vi "_Check Voltages.vi"(6 "Unit":bool, 7 "SGInput":dbl[](array[numeric]), 8 "ADC Table":T3[](array[typedef]), 9 "ADC Values":i32[](array[numeric]), 10 "VoltageInput":dbl[](array[numeric]), 11 "Reference":T1) -> (0 "Source 2 Type:":T2 items=["None", "ESI", "APCI", "APPI", "MicroSpray"], 1 "Source 1 Type:":T2 items=["None", "ESI", "APCI", "APPI", "MicroSpray"], 2 "SVG OK":bool, 3 "Voltage OK":bool, 4 "Pressure":string[][](array[string]), 5 "DC OK":bool)   [LabVIEW 2018]
uses:
  Type/_RT Configuration 2.ctl
  Type/_Source Type.ctl
  Type/_Model Family.ctl
  <vilib>/Utility/miscctls.llb/LVRowAndColumnTypeDef.ctl
  Configuration/_Global Configuration.vi
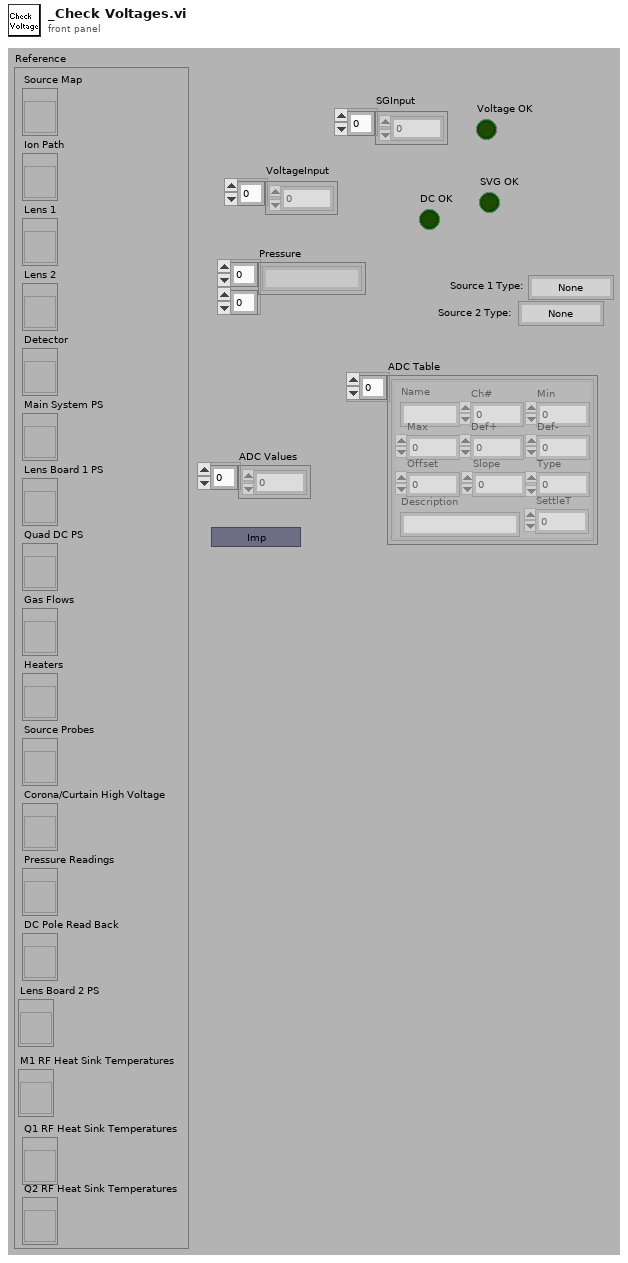
[diagram p1: front panel]
types:
  T1 = cluster{"Source Map":refnum<vi>, "Ion Path":refnum<vi>, "Lens 1":refnum<vi>, "Lens 2":refnum<vi>, "Detector":refnum<vi>, "Main System PS":refnum<vi>, "Lens Board 1 PS":refnum<vi>, "Quad DC PS":refnum<vi>, "Gas Flows":refnum<vi>, "Heaters":refnum<vi>, "Source Probes":refnum<vi>, "Corona/Curtain High Voltage":refnum<vi>, "Pressure Readings":refnum<vi>, "DC Pole Read Back":refnum<vi>, "Lens Board 2 PS":refnum<vi>, "M1 RF Heat Sink Temperatures":refnum<vi>, "Q1 RF Heat Sink Temperatures":refnum<vi>, "Q2 RF Heat Sink Temperatures":refnum<vi>}
  T2 = typedef "_Source Type.ctl" = i8
  T3 = typedef "_RT Configuration 2.ctl" = cluster{"Name":string, "Ch#":u8, "Min":dbl, "Max":dbl, "Def+":dbl, "Def-":dbl, "Offset":dbl, "Slope":dbl, "Type":u8, "Description":string, "SettleT":dbl}
  T4 = typedef "LVRowAndColumnTypeDef.ctl" = cluster{"Row":i32, "Column":i32}
  T5 = typedef "_Model Family.ctl" = u16
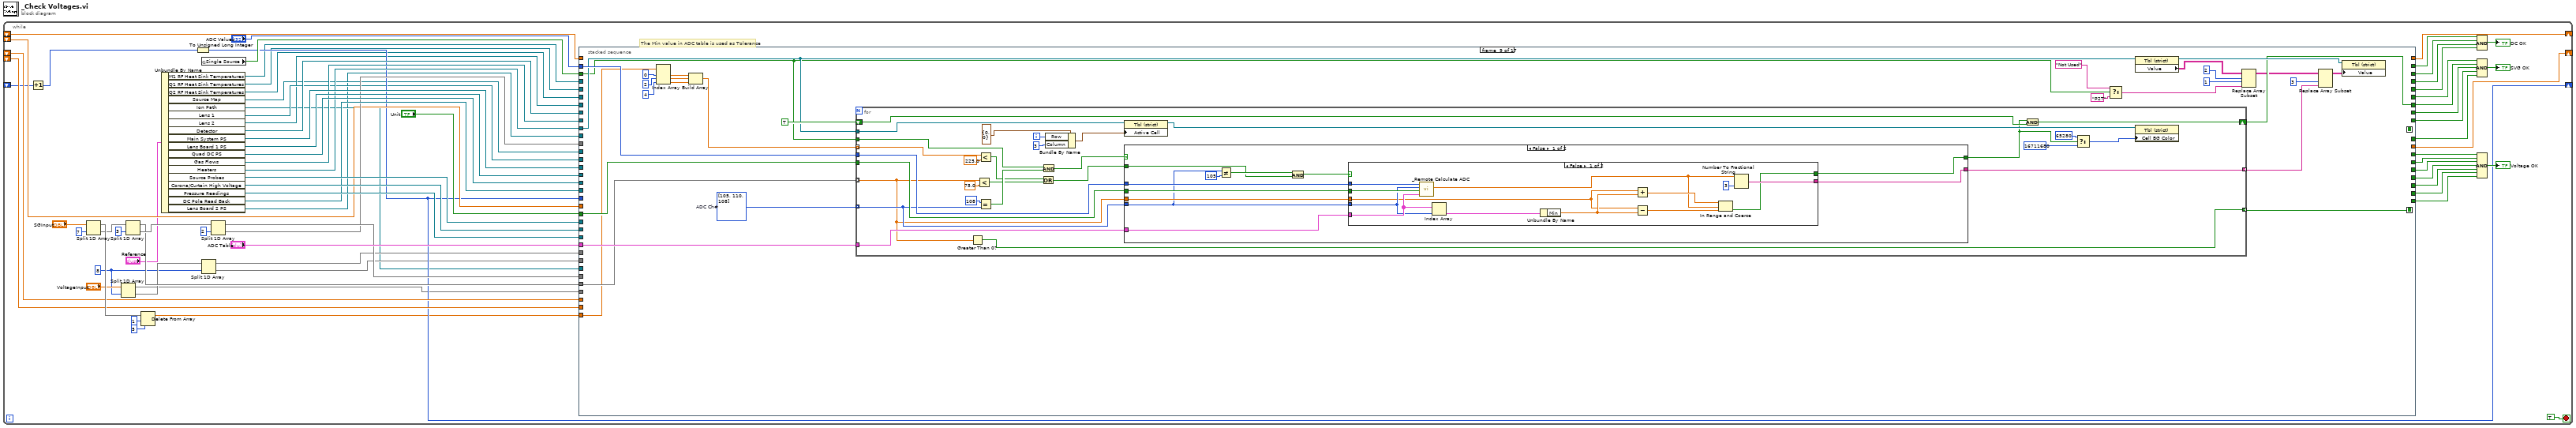
[diagram p0: block diagram]
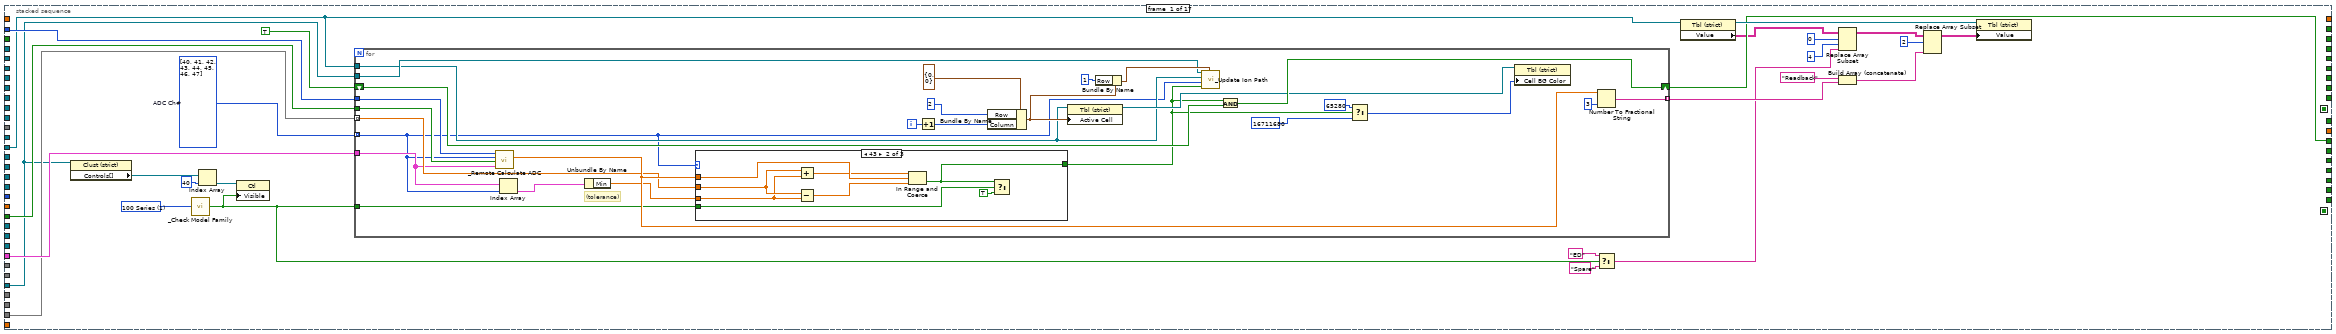
[diagram p2: hidden frame]
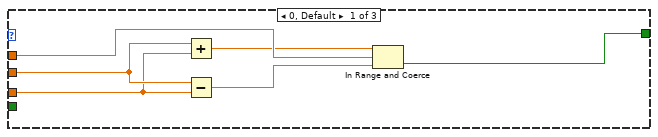
[diagram p3: hidden frame]
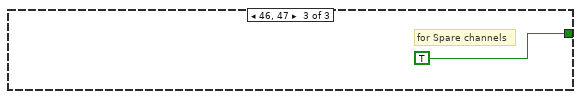
[diagram p4: hidden frame]
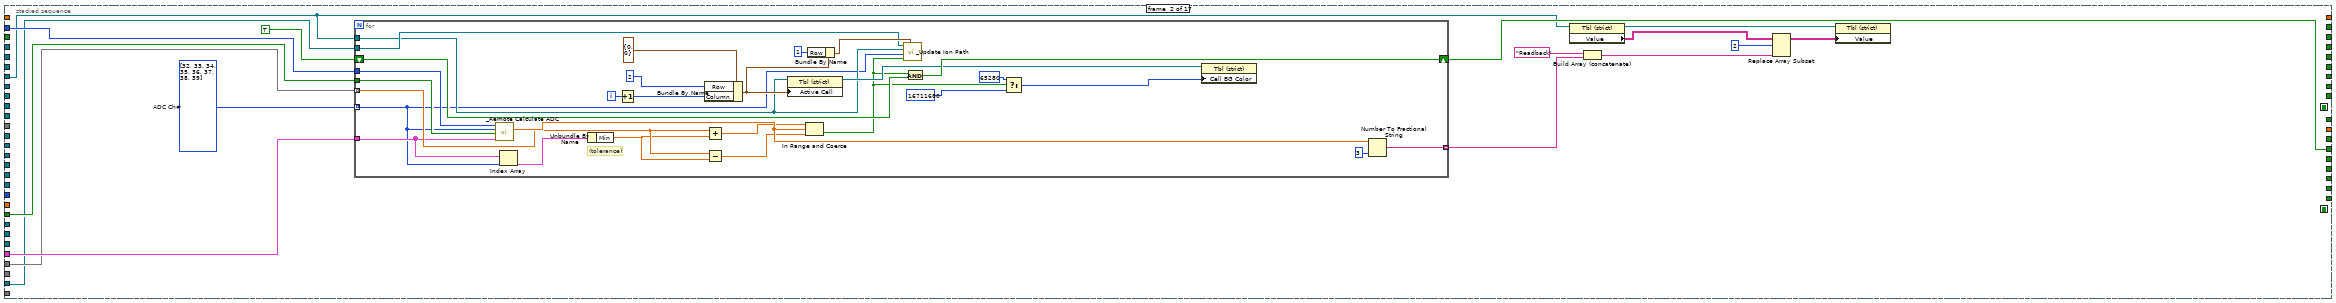
[diagram p5: hidden frame]
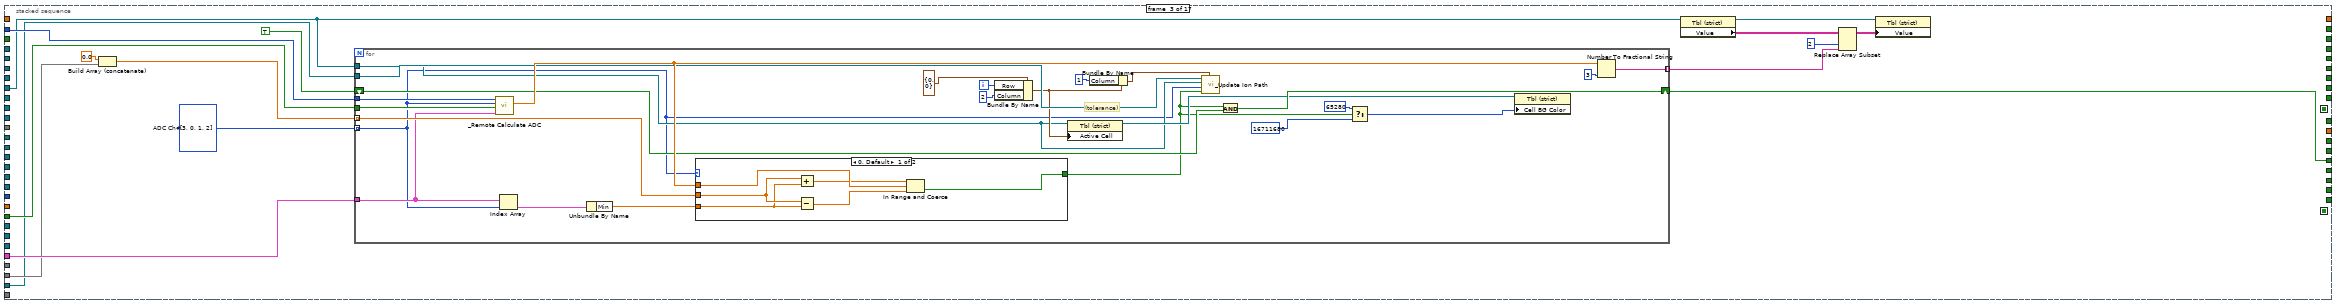
[diagram p6: hidden frame]
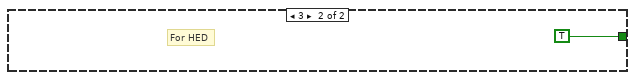
[diagram p7: hidden frame]
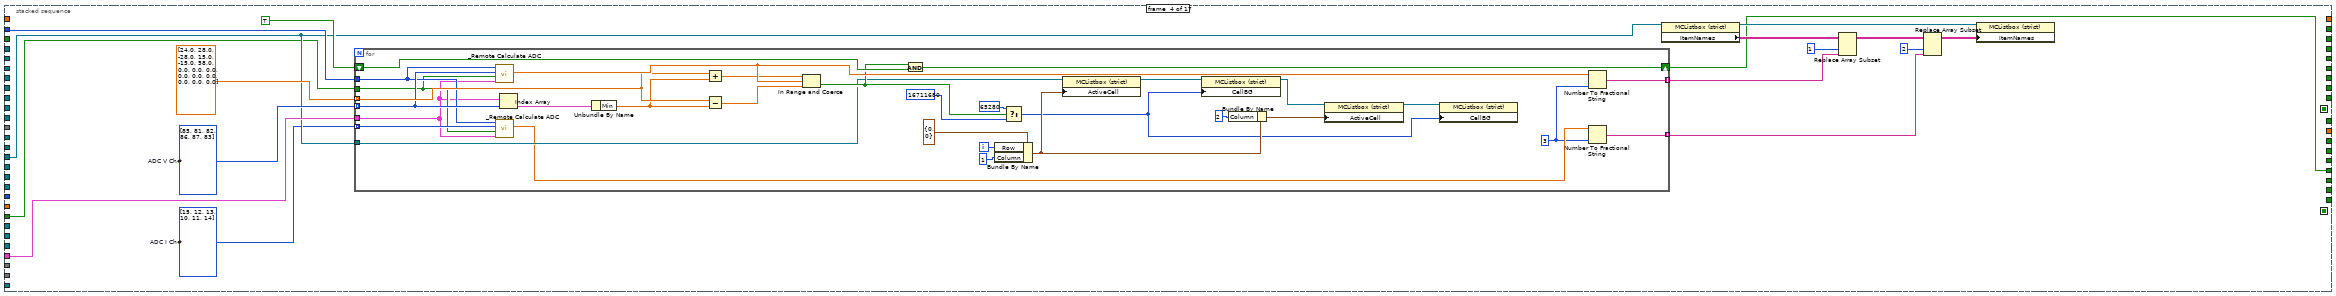
[diagram p8: hidden frame]
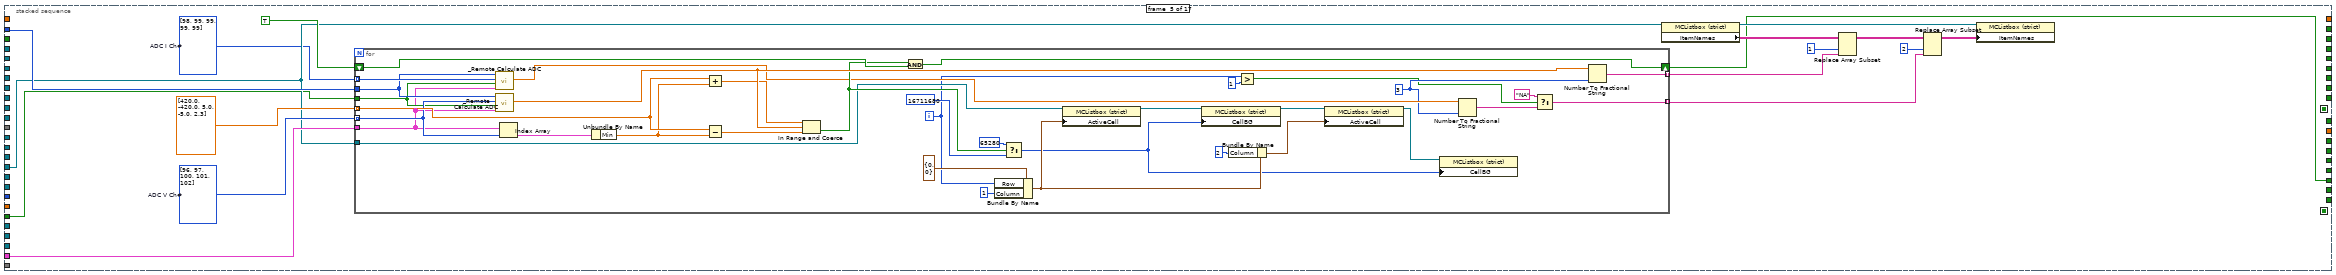
[diagram p9: hidden frame]
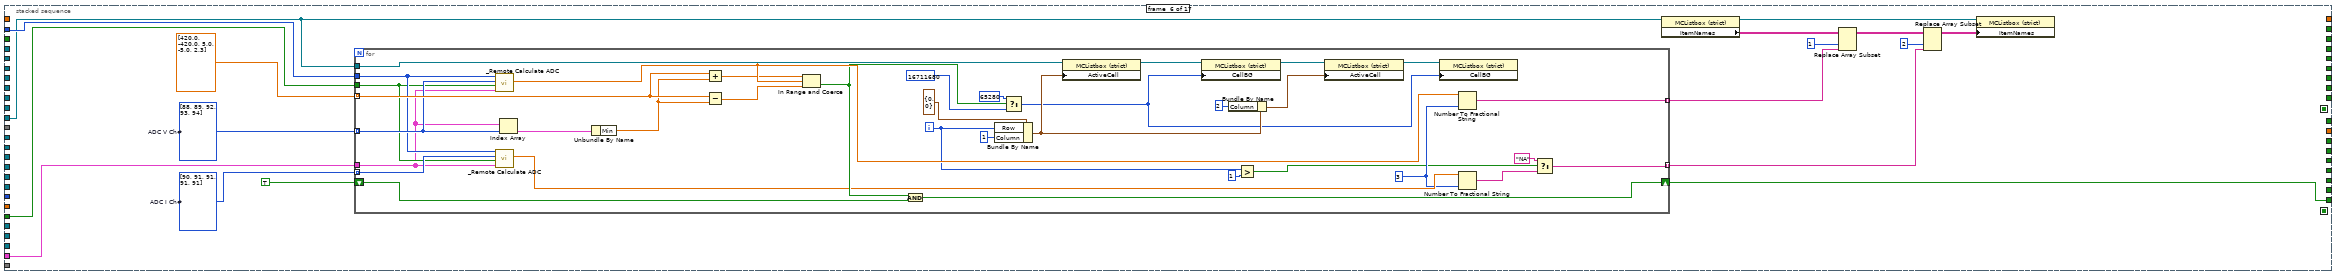
[diagram p10: hidden frame]
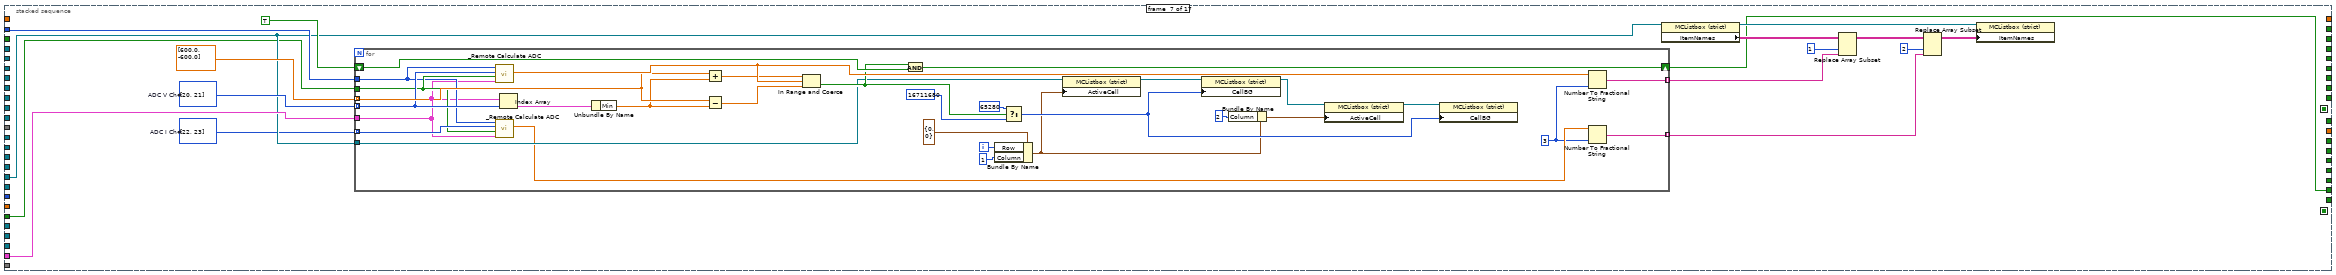
[diagram p11: hidden frame]
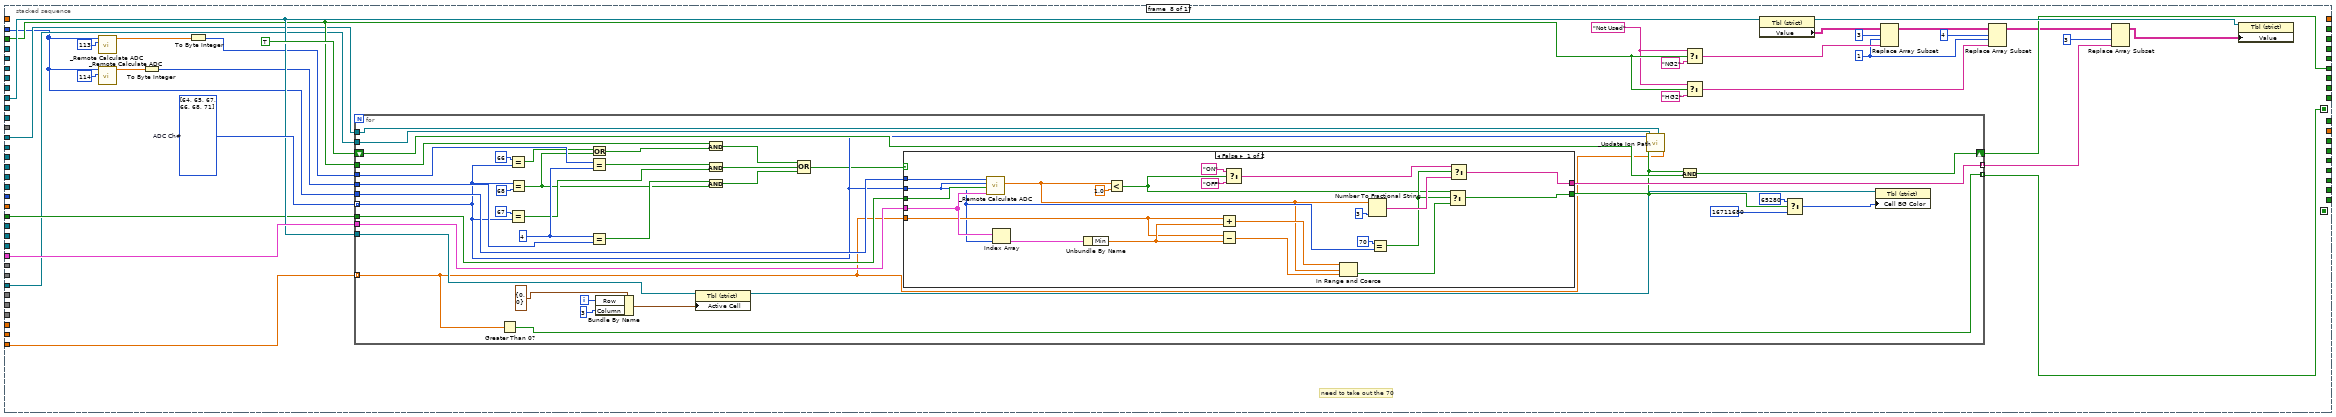
[diagram p12: hidden frame]
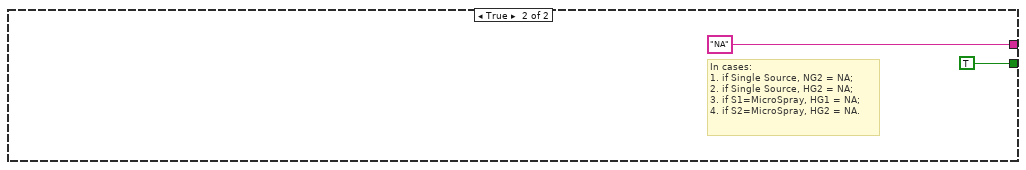
[diagram p13: hidden frame]
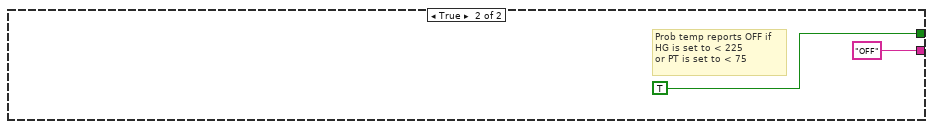
[diagram p14: hidden frame]
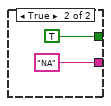
[diagram p15: hidden frame]
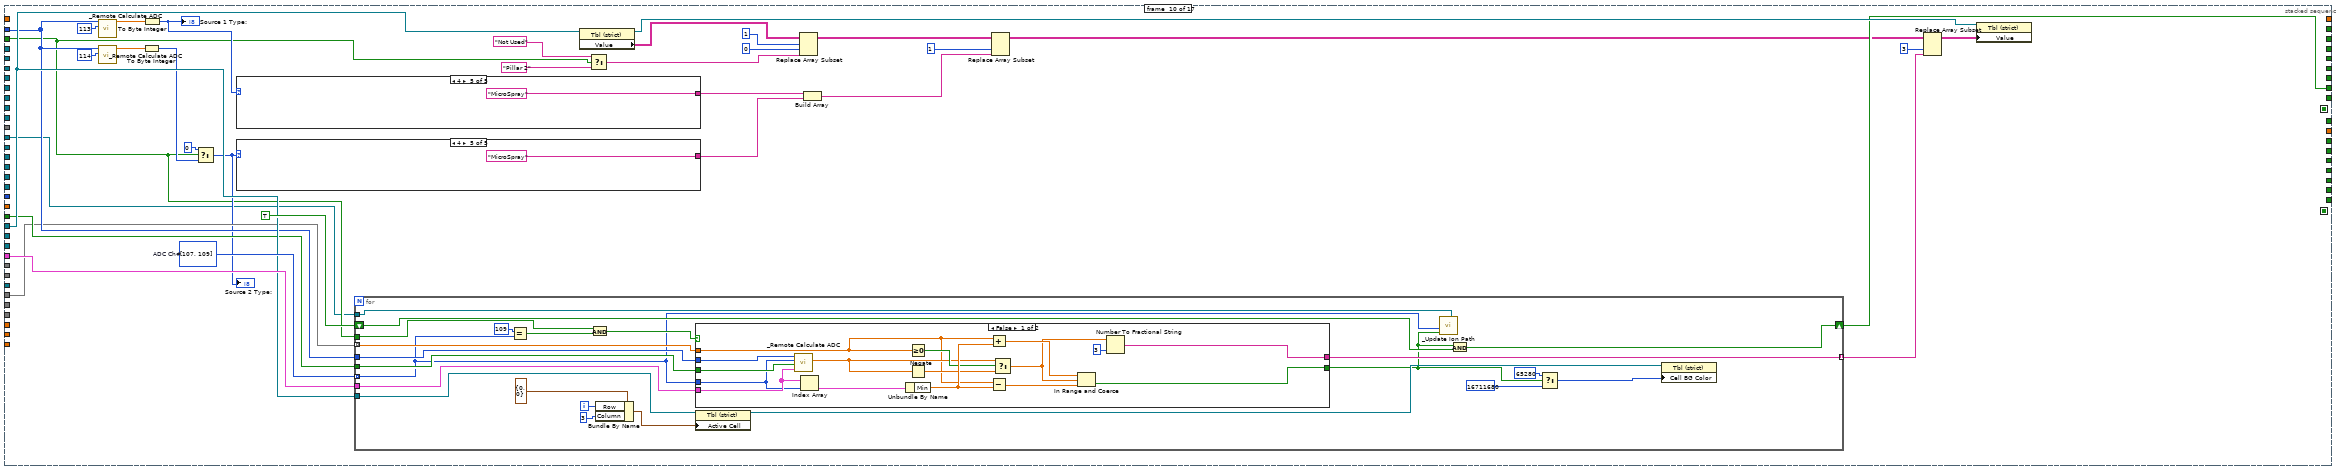
[diagram p16: hidden frame]
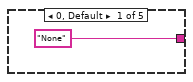
[diagram p17: hidden frame]
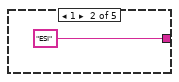
[diagram p18: hidden frame]
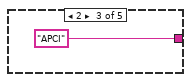
[diagram p19: hidden frame]
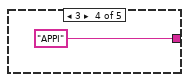
[diagram p20: hidden frame]
diagram:
  n1 = while {
    shift-right: [w35] -> _
    shift-left: _ -> [w34]
    shift-left: _ -> [w31]
    shift-right: [w33] -> _
    shift-left: _ -> [w32]
    shift-left: _ -> [w30]
    shift-right: [w27] -> _
    shift-left: _ -> [w29]
    stop <- TRUE stop-if-true
    w21 = 8 ("index")
    # "The Min value in ADC table is used as Tolerance"
    n2 = Increment(x=w29) -> (x+1=w28:u32)
    n3 = Split 1D Array(array="SGInput", index=7) -> (first subarray=w45:dbl[], second subarray=w43:dbl[])
    n4 = Split 1D Array(array="VoltageInput", index=w21) -> (first subarray=w20:dbl[], second subarray=w23:dbl[])
    n5 = Split 1D Array(array=w43, index=3) -> (first subarray=w40:dbl[], second subarray=w41:dbl[])
    n6 = Delete From Array(array=w45, length=1, index=5) -> (array with subset deleted=w3:dbl[])  [unwired: 1 out]
    n7 = Unbundle By Name("Reference") -> ("M1 RF Heat Sink Temperatures"=w11:refnum<vi>, "Q1 RF Heat Sink Temperatures"=w10:refnum<vi>, "Q2 RF Heat Sink Temperatures"=w9:refnum<vi>, "Source Map"=w15:refnum<vi>, "Ion Path"=w16:refnum<vi>, "Lens 1"=w26:refnum<vi>, "Lens 2"=w25:refnum<vi>, "Detector"=w71:refnum<vi>, "Main System PS"=w70:refnum<vi>, "Lens Board 1 PS"=w69:refnum<vi>, "Quad DC PS"=w68:refnum<vi>, "Gas Flows"=w60:refnum<vi>, "Heaters"=w59:refnum<vi>, "Source Probes"=w58:refnum<vi>, "Corona/Curtain High Voltage"=w57:refnum<vi>, "Pressure Readings"=w56:refnum<vi>, "DC Pole Read Back"=w49:refnum<vi>, "Lens Board 2 PS"=w13:refnum<vi>)
    n8 = To Unsigned Long Integer(number=w28) -> (unsigned 32bit integer=w27:u32)
    n9 = global read "_Global Configuration.vi" "Single Source"() -> (w37:bool)
    n10 = Split 1D Array(array=w23, index=w21) -> (first subarray=w19:dbl[], second subarray=w18:dbl[])
    n11 = Split 1D Array(array=w41, index=2) -> (first subarray=w39:dbl[], second subarray=w38:dbl[])
    n12 = stacked-sequence {
      seq-local: [_ _ _ _ _ _ _ _ w528 _ _ _ _ _ _ _ _] -> [_ _ _ _ _ _ _ _ _ _ _ _ _ _ _ _ w955]
      seq-local: [_ _ _ _ _ _ _ w443 _ _ _ _ _ _ _ _ _] -> [_ _ _ _ _ _ _ _ _ _ _ _ _ _ _ _ w952]
      tunnel: w71 -> [_ _ w196 _ _ _ _ _ _ _ _ _ _ _ _ _ _]
      tunnel: w70 -> [_ _ _ w240 _ _ _ _ _ _ _ _ _ _ _ _ _]
      tunnel: w69 -> [_ _ _ _ w288 _ _ _ _ _ _ _ _ _ _ _ _]
      tunnel: w68 -> [_ _ _ _ _ _ w392 _ _ _ _ _ _ _ _ _ _]
      tunnel: "ADC Values" -> [w97 w155 w199 w247 w295 w347 w399 w436 w555 w638 w713 w765 w830 w859 w890 w921 _]
      tunnel: "ADC Table" -> [w96 w154 w198 w246 w294 w346 w398 w464 w554 w646 w712 w764 w829 w858 w889 w920 _]
      tunnel: [_ _ w190 _ _ _ _ _ _ _ _ _ _ _ _ _ _] -> w65
      tunnel: [_ _ _ w239 _ _ _ _ _ _ _ _ _ _ _ _ _] -> w64
      tunnel: [_ _ _ _ w287 _ _ _ _ _ _ _ _ _ _ _ _] -> w63
      tunnel: [_ _ _ _ _ _ w391 _ _ _ _ _ _ _ _ _ _] -> w62
      tunnel: w60 -> [_ _ _ _ _ _ _ w459 _ _ _ _ _ _ _ _ _]
      tunnel: [_ _ _ _ _ _ _ w458 _ _ _ _ _ _ _ _ _] -> w55
      tunnel: w59 -> [_ _ _ _ _ _ _ _ w548 _ _ _ _ _ _ _ _]
      tunnel: [_ _ _ _ _ _ _ _ w547 _ _ _ _ _ _ _ _] -> w54
      tunnel: w58 -> [_ _ _ _ _ _ _ _ _ w642 _ _ _ _ _ _ _]
      tunnel: [_ _ _ _ _ _ _ _ _ w641 _ _ _ _ _ _ _] -> w53
      tunnel: w57 -> [_ _ _ _ _ _ _ _ _ _ w707 _ _ _ _ _ _]
      tunnel: [_ _ _ _ _ _ _ _ _ _ w706 _ _ _ _ _ _] -> w52
      tunnel: w56 -> [_ _ _ _ _ _ _ _ _ _ _ w760 _ _ _ _ _]
      tunnel: [_ _ _ _ _ _ _ _ _ _ _ w761 _ _ _ _ _] -> w51
      tunnel: [_ _ _ _ _ _ _ _ _ _ _ _ w824 _ _ _ _] -> w8
      tunnel: w49 -> [_ _ _ _ _ _ _ _ _ _ _ _ w821 _ _ _ _]
      tunnel: "Unit" -> [w92 w149 w189 w238 w286 w340 w390 w457 w546 w631 w705 w757 w823 w853 w884 w916 _]
      tunnel: w3 -> [_ _ _ _ _ _ _ w456 w536 _ _ _ _ _ _ _ _]
      tunnel: w40 -> [_ _ _ _ _ _ _ _ w545 _ _ _ _ _ _ _ _]
      tunnel: w39 -> [_ _ _ _ _ _ _ _ _ w626 _ _ _ _ _ _ _]
      tunnel: w38 -> [_ _ _ _ _ _ _ _ _ _ w702 _ _ _ _ _ _]
      tunnel: w37 -> [_ _ _ _ _ _ _ w455 w538 w615 _ _ _ _ _ _ _]
      tunnel: [_ _ _ _ _ _ _ _ _ _ _ w755 _ _ _ _ _] -> w35
      tunnel: w34 -> [_ _ _ _ _ _ _ _ _ _ _ w754 _ _ _ _ _]
      tunnel: [_ _ _ _ _ _ _ _ _ _ _ w753 _ _ _ _ _] -> w33
      tunnel: w32 -> [_ _ _ _ _ _ _ _ _ _ _ w752 _ _ _ _ _]
      tunnel: w31 -> [_ _ _ _ _ _ _ _ _ _ _ w751 _ _ _ _ _]
      tunnel: w30 -> [_ _ _ _ _ _ _ _ _ _ _ w750 _ _ _ _ _]
      tunnel: w27 -> [_ _ _ _ _ _ _ _ _ _ _ w747 _ _ _ _ _]
      tunnel: w26 -> [w91 _ _ _ _ _ _ _ _ _ _ _ _ _ _ _ _]
      tunnel: w25 -> [_ w142 _ _ _ _ _ _ _ _ _ _ _ _ _ _ _]
      tunnel: [w86 _ _ _ _ _ _ _ _ _ _ _ _ _ _ _ _] -> w24
      tunnel: w20 -> [w85 _ _ _ _ _ _ _ _ _ _ _ _ _ _ _ _]
      tunnel: w19 -> [_ w143 _ _ _ _ _ _ _ _ _ _ _ _ _ _ _]
      tunnel: w18 -> [_ _ w187 _ _ _ _ _ _ _ _ _ _ _ _ _ _]
      tunnel: [_ w144 _ _ _ _ _ _ _ _ _ _ _ _ _ _ _] -> w17
      tunnel: w16 -> [w75 w141 w185 _ _ _ _ w441 _ _ w700 _ _ _ _ _ _]
      tunnel: w15 -> [_ _ _ _ _ _ _ w442 _ w614 w699 _ _ _ _ _ w958]
      tunnel: w13 -> [_ _ _ _ _ w334 _ _ _ _ _ _ _ _ _ _ _]
      tunnel: [_ _ _ _ _ w333 _ _ _ _ _ _ _ _ _ _ _] -> w12
      tunnel: w11 -> [_ _ _ _ _ _ _ _ _ _ _ _ _ w850 _ _ _]
      tunnel: w10 -> [_ _ _ _ _ _ _ _ _ _ _ _ _ _ w881 _ _]
      tunnel: w9 -> [_ _ _ _ _ _ _ _ _ _ _ _ _ _ _ w913 _]
      tunnel: [_ _ _ _ _ _ _ _ _ _ _ _ _ w849 _ _ _] -> w6
      tunnel: [_ _ _ _ _ _ _ _ _ _ _ _ _ _ w880 _ _] -> w5
      tunnel: [_ _ _ _ _ _ _ _ _ _ _ _ _ _ _ w911 _] -> w4
      frame #0 {
        w77 = T5 1 items=["8080 Series", "100 Series", "200 Series", "300 Series", "Other Series"] ("Model Family (100)")
        w98 = u8[] [40, 41, 42, 43, 44, 45, 46, 47]  # ADC Ch#
        n13 = property class="Clust (strict)"(reference=w75) -> ("Controls[]"=w76:refnum<vi>[])  [unwired: 1 in, 2 out]
        n14 = call "_Check Model Family.vi"("Model Family (100)"=w77) -> ("Yes"=w72:bool)
        n15 = Index Array(array=w76, index=40) -> (element=w73:refnum<vi>)
        n16 = property class="Ctl"(reference=w73, "Visible"=w72) -> ()  [unwired: 1 in, 2 out]
        n17 = for {
          tunnel: w98 -> [w100] mode=indexing
          tunnel: w85 -> [w122] mode=indexing
          tunnel: w97 -> [w125]
          tunnel: w96 -> [w112]
          shift-right: [w120] -> w86
          shift-left: TRUE -> [w121]
          tunnel: w91 -> [w101]
          tunnel: [w114] -> w88 mode=indexing
          tunnel: w92 -> [w113]
          tunnel: w75 -> [w102]
          tunnel: w72 -> [w99]
          i -> [w108]
          # "(tolerance)"
          n18 = call "_Remote Calculate ADC.vi"("ADC Table"=w112, "Unit"=w113, "ADC Channel (64)"=w100, "ADC Values"=w125) -> ("User Value"=w123:dbl)  [unwired: 3 out]
          n19 = Index Array(array=w112, index=w100) -> (element=w111:T3)
          n20 = Unbundle By Name(w111) -> ("Min"=w110:dbl)
          n21 = case shown="43" w100 {
            tunnel: w123 -> [w131 w139 _]
            tunnel: w122 -> [w130 w138 _]
            tunnel: [w129 w133 TRUE] -> w106
            tunnel: w110 -> [w126 w135 _]
            tunnel: w99 -> [_ w134 _]
            frame 0, Default {
              n22 = Add(x=w130, y=w126) -> (x+y=w128:dbl)
              n23 = Subtract(x=w130, y=w126) -> (x-y=w127:dbl)
              n24 = In Range and Coerce(upper limit=w128, x=w131, lower limit=w127) -> (In Range?=w129:bool)  [unwired: 1 out]
            }
            frame 43 {
              n25 = Add(x=w138, y=w135) -> (x+y=w137:dbl)
              n26 = Subtract(x=w138, y=w135) -> (x-y=w136:dbl)
              n27 = In Range and Coerce(upper limit=w137, x=w139, lower limit=w136) -> (In Range?=w133:bool)  [unwired: 1 out]
              n28 = Select(t=w133, s=w134, f=TRUE) -> ()  [unwired: 1 out]
            }
            frame 46, 47 {
              # "for Spare channels"
            }
          }
          n29 = Increment(x=w108) -> (x+1=w107:i32)
          n30 = Bundle By Name(cluster=T4 {"Row"=0, "Column"=0} ("Active Cell:Active Cell"), "Row"=2 ("Column"), "Column"=w107) -> (w105:T4)
          n31 = property class="Tbl (strict)"(reference=w101, "Active Cell"=w105) -> (reference out=w116:refnum<vi>)  [unwired: 1 in, 1 out]
          n32 = Bundle By Name(cluster=w105, "Row"=1) -> (w104:T4)
          n33 = call "_Update Ion Path.vi"("Current Cell"=w104, "Voltage OK"=w106, "ADC Ch#"=w100, "Lens Table"=w101, "Ion Path"=w102) -> ()  [unwired: 2 in, 3 out]
          n34 = And(x=w106, y=w121) -> (x .and. y?=w120:bool)
          n35 = Select(t=u32 65280 ("Active Cell:Cell Background Color"), s=w106, f=u32 16711680 ("Active Cell:Cell Background Color")) -> (s? t:f=w115:u32)
          n36 = property class="Tbl (strict)"(reference=w116, "Cell BG Color"=w115) -> ()  [unwired: 1 in, 2 out]
          n37 = Number To Fractional String(number=w123, precision (6)=i16 3) -> (F-format string=w114:string)  [unwired: 2 out]
        }
        n38 = Select(t="ED", s=w72, f="Spare") -> (s? t:f=w78:string)
        n39 = property class="Tbl (strict)"(reference=w91) -> (reference out=w94:refnum<vi>, "Value"=w82:string[][])  [unwired: 1 in, 1 out]
        n40 = Replace Array Subset(array=w82, new element=w78, index (row)=0, index (col)=4 ("disabled index (col)")) -> (w81:string[][])
        n41 = Build Array (concatenate)("Readback", w88) -> (w87:string[])
        n42 = Replace Array Subset(array=w81, new element=w87, index (row)=2 ("disabled index (col)")) -> (w93:string[][])  [unwired: 1 in]
        n43 = property class="Tbl (strict)"(reference=w94, "Value"=w93) -> ()  [unwired: 1 in, 2 out]
      }
      frame #1 {
        w156 = u8[] [32, 33, 34, 35, 36, 37, 38, 39]  # ADC Ch#
        n44 = for {
          tunnel: w156 -> [w157] mode=indexing
          tunnel: w143 -> [w181] mode=indexing
          tunnel: w155 -> [w184]
          tunnel: w154 -> [w171]
          shift-right: [w179] -> w144
          shift-left: TRUE -> [w180]
          tunnel: w142 -> [w158]
          tunnel: [w173] -> w146 mode=indexing
          tunnel: w149 -> [w172]
          tunnel: w141 -> [w159]
          i -> [w167]
          # "(tolerance)"
          n45 = call "_Remote Calculate ADC.vi"("ADC Table"=w171, "Unit"=w172, "ADC Channel (64)"=w157, "ADC Values"=w184) -> ("User Value"=w182:dbl)  [unwired: 3 out]
          n46 = Index Array(array=w171, index=w157) -> (element=w170:T3)
          n47 = Unbundle By Name(w170) -> ("Min"=w169:dbl)
          n48 = Increment(x=w167) -> (x+1=w166:i32)
          n49 = Bundle By Name(cluster=T4 {"Row"=0, "Column"=0} ("Active Cell:Active Cell"), "Row"=2 ("Column"), "Column"=w166) -> (w161:T4)
          n50 = Add(x=w181, y=w169) -> (x+y=w165:dbl)
          n51 = Subtract(x=w181, y=w169) -> (x-y=w164:dbl)
          n52 = property class="Tbl (strict)"(reference=w158, "Active Cell"=w161) -> (reference out=w175:refnum<vi>)  [unwired: 1 in, 1 out]
          n53 = In Range and Coerce(upper limit=w165, x=w182, lower limit=w164) -> (In Range?=w163:bool)  [unwired: 1 out]
          n54 = Bundle By Name(cluster=w161, "Row"=1) -> (w160:T4)
          n55 = call "_Update Ion Path.vi"("Current Cell"=w160, "Voltage OK"=w163, "ADC Ch#"=w157, "Lens Table"=w158, "Ion Path"=w159) -> ()  [unwired: 2 in, 3 out]
          n56 = And(x=w163, y=w180) -> (x .and. y?=w179:bool)
          n57 = Select(t=u32 65280 ("Active Cell:Cell Background Color"), s=w163, f=u32 16711680 ("Active Cell:Cell Background Color")) -> (s? t:f=w174:u32)
          n58 = property class="Tbl (strict)"(reference=w175, "Cell BG Color"=w174) -> ()  [unwired: 1 in, 2 out]
          n59 = Number To Fractional String(number=w182, precision (6)=i16 3) -> (F-format string=w173:string)  [unwired: 2 out]
        }
        n60 = property class="Tbl (strict)"(reference=w142) -> (reference out=w152:refnum<vi>, "Value"=w151:string[][])  [unwired: 1 in, 1 out]
        n61 = Build Array (concatenate)("Readback", w146) -> (w145:string[])
        n62 = Replace Array Subset(array=w151, new element=w145, index (row)=2 ("disabled index (col)")) -> (w150:string[][])  [unwired: 1 in]
        n63 = property class="Tbl (strict)"(reference=w152, "Value"=w150) -> ()  [unwired: 1 in, 2 out]
      }
      frame #2 {
        w200 = u8[] [3, 0, 1, 2]  # ADC Ch#
        n64 = Build Array (concatenate)(0.0 ("element"), w187) -> (w186:dbl[])
        n65 = for {
          tunnel: w200 -> [w201] mode=indexing
          tunnel: w186 -> [w222] mode=indexing
          tunnel: w199 -> [w225]
          tunnel: w198 -> [w211]
          shift-right: [w220] -> w190
          shift-left: TRUE -> [w221]
          tunnel: w196 -> [w202]
          tunnel: [w213] -> w192 mode=indexing
          tunnel: w189 -> [w212]
          tunnel: w185 -> [w206]
          i -> [w210]
          # "(tolerance)"
          n66 = call "_Remote Calculate ADC.vi"("ADC Table"=w211, "Unit"=w212, "ADC Channel (64)"=w201, "ADC Values"=w225) -> ("User Value"=w223:dbl)  [unwired: 3 out]
          n67 = Index Array(array=w211, index=w201) -> (element=w209:T3)
          n68 = Unbundle By Name(w209) -> ("Min"=w208:dbl)
          n69 = case shown="0, Default" w201 {
            tunnel: w223 -> [w231 _]
            tunnel: w222 -> [w230 _]
            tunnel: [w229 TRUE] -> w207
            tunnel: w208 -> [w226 _]
            frame 0, Default {
              n70 = Add(x=w230, y=w226) -> (x+y=w228:dbl)
              n71 = Subtract(x=w230, y=w226) -> (x-y=w227:dbl)
              n72 = In Range and Coerce(upper limit=w228, x=w231, lower limit=w227) -> (In Range?=w229:bool)  [unwired: 1 out]
            }
            frame 3 {
              # "For HED"
            }
          }
          n73 = Bundle By Name(cluster=T4 {"Row"=0, "Column"=0} ("Active Cell:Active Cell"), "Row"=w210, "Column"=2) -> (w204:T4)
          n74 = property class="Tbl (strict)"(reference=w202, "Active Cell"=w204) -> (reference out=w215:refnum<vi>)  [unwired: 1 in, 1 out]
          n75 = Bundle By Name(cluster=w204, "Column"=1 ("Row")) -> (w203:T4)
          n76 = call "_Update Ion Path.vi"("Current Cell"=w203, "Voltage OK"=w207, "ADC Ch#"=w201, "Lens Table"=w202, "Ion Path"=w206) -> ()  [unwired: 2 in, 3 out]
          n77 = And(x=w207, y=w221) -> (x .and. y?=w220:bool)
          n78 = Select(t=u32 65280 ("Active Cell:Cell Background Color"), s=w207, f=u32 16711680 ("Active Cell:Cell Background Color")) -> (s? t:f=w214:u32)
          n79 = property class="Tbl (strict)"(reference=w215, "Cell BG Color"=w214) -> ()  [unwired: 1 in, 2 out]
          n80 = Number To Fractional String(number=w223, precision (6)=i16 3) -> (F-format string=w213:string)  [unwired: 2 out]
        }
        n81 = property class="Tbl (strict)"(reference=w196) -> (reference out=w195:refnum<vi>, "Value"=w194:string[][])  [unwired: 1 in, 1 out]
        n82 = Replace Array Subset(array=w194, new element=w192, index (col)=2 ("disabled index (col)")) -> (w191:string[][])  [unwired: 1 in]
        n83 = property class="Tbl (strict)"(reference=w195, "Value"=w191) -> ()  [unwired: 1 in, 2 out]
      }
      frame #3 {
        w237 = u8[] [15, 12, 13, 10, 11, 14]  # ADC I Ch#
        w249 = u8[] [85, 81, 82, 86, 87, 83]  # ADC V Ch#
        n84 = for {
          tunnel: w249 -> [w264] mode=indexing
          tunnel: dbl[] [24.0, 28.0, -28.0, 15.0, -15.0, 58.0, 0.0, 0.0, 0.0, 0.0, 0.0, 0.0, 0.0, 0.0, 0.0] ("VoltageInput 2") -> [w279] mode=indexing
          tunnel: w247 -> [w261]
          tunnel: w246 -> [w259]
          shift-right: [w277] -> w239
          shift-left: TRUE -> [w278]
          tunnel: w240 -> [w270]
          tunnel: [w268] -> w241 mode=indexing
          tunnel: w238 -> [w260]
          tunnel: w237 -> [w262] mode=indexing
          tunnel: [w256] -> w233 mode=indexing
          i -> [w271]
          w257 = i16 3 ("precision (6)")
          n85 = call "_Remote Calculate ADC.vi"("ADC Table"=w259, "Unit"=w260, "ADC Channel (64)"=w264, "ADC Values"=w261) -> ("User Value"=w280:dbl)  [unwired: 3 out]
          n86 = call "_Remote Calculate ADC.vi"("ADC Table"=w259, "Unit"=w260, "ADC Channel (64)"=w262, "ADC Values"=w261) -> ("User Value"=w258:dbl)  [unwired: 3 out]
          n87 = Index Array(array=w259, index=w264) -> (element=w265:T3)
          n88 = Unbundle By Name(w265) -> ("Min"=w263:dbl)
          n89 = Add(x=w279, y=w263) -> (x+y=w267:dbl)
          n90 = Subtract(x=w279, y=w263) -> (x-y=w266:dbl)
          n91 = In Range and Coerce(upper limit=w267, x=w280, lower limit=w266) -> (In Range?=w275:bool)  [unwired: 1 out]
          n92 = And(x=w275, y=w278) -> (x .and. y?=w277:bool)
          n93 = Bundle By Name(cluster=T4 {"Row"=0, "Column"=0} ("Active Cell:Active Cell"), "Row"=w271, "Column"=1) -> (w253:T4)
          n94 = Select(t=u32 65280 ("Active Cell:Cell Background Color"), s=w275, f=u32 16711680 ("Active Cell:Cell Background Color")) -> (s? t:f=w250:u32)
          n95 = property class="MCListbox (strict)"(reference=w270, "ActiveCell"=w253) -> (reference out=w269:refnum<vi>)  [unwired: 1 in, 1 out]
          n96 = property class="MCListbox (strict)"(reference=w269, "CellBG"=w250) -> (reference out=w254:refnum<vi>)  [unwired: 1 in, 1 out]
          n97 = Bundle By Name(cluster=w253, "Column"=2) -> (w251:T4)
          n98 = property class="MCListbox (strict)"(reference=w254, "ActiveCell"=w251) -> (reference out=w255:refnum<vi>)  [unwired: 1 in, 1 out]
          n99 = property class="MCListbox (strict)"(reference=w255, "CellBG"=w250) -> ()  [unwired: 1 in, 2 out]
          n100 = Number To Fractional String(number=w280, precision (6)=w257) -> (F-format string=w268:string)  [unwired: 2 out]
          n101 = Number To Fractional String(number=w258, precision (6)=w257) -> (F-format string=w256:string)  [unwired: 2 out]
        }
        n102 = property class="MCListbox (strict)"(reference=w240) -> (reference out=w244:refnum<vi>, "ItemNames"=w243:string[][])  [unwired: 1 in, 1 out]
        n103 = Replace Array Subset(array=w243, new element=w241, index (col)=1 ("disabled index (col)")) -> (w236:string[][])  [unwired: 1 in]
        n104 = Replace Array Subset(array=w236, new element=w233, index (col)=2 ("disabled index (col)")) -> (w235:string[][])  [unwired: 1 in]
        n105 = property class="MCListbox (strict)"(reference=w244, "ItemNames"=w235) -> ()  [unwired: 1 in, 2 out]
      }
      frame #4 {
        w282 = u8[] [98, 99, 99, 99, 99]  # ADC I Ch#
        w297 = u8[] [96, 97, 100, 101, 102]  # ADC V Ch#
        n106 = for {
          tunnel: w297 -> [w316] mode=indexing
          tunnel: dbl[] [420.0, -420.0, 5.0, -5.0, 2.3] ("VoltageInput 2") -> [w331] mode=indexing
          tunnel: w295 -> [w314]
          tunnel: w294 -> [w312]
          shift-right: [w329] -> w287
          shift-left: TRUE -> [w330]
          tunnel: w288 -> [w323]
          tunnel: [w321] -> w289 mode=indexing
          tunnel: w286 -> [w313]
          tunnel: w282 -> [w315] mode=indexing
          tunnel: [w304] -> w281 mode=indexing
          i -> [w309]
          w310 = i16 3 ("precision (6)")
          n107 = call "_Remote Calculate ADC.vi"("ADC Table"=w312, "Unit"=w313, "ADC Channel (64)"=w315, "ADC Values"=w314) -> ("User Value"=w311:dbl)  [unwired: 3 out]
          n108 = call "_Remote Calculate ADC.vi"("ADC Table"=w312, "Unit"=w313, "ADC Channel (64)"=w316, "ADC Values"=w314) -> ("User Value"=w332:dbl)  [unwired: 3 out]
          n109 = Index Array(array=w312, index=w316) -> (element=w318:T3)
          n110 = Unbundle By Name(w318) -> ("Min"=w317:dbl)
          n111 = Add(x=w331, y=w317) -> (x+y=w320:dbl)
          n112 = Subtract(x=w331, y=w317) -> (x-y=w319:dbl)
          n113 = In Range and Coerce(upper limit=w320, x=w332, lower limit=w319) -> (In Range?=w327:bool)  [unwired: 1 out]
          n114 = And(x=w327, y=w330) -> (x .and. y?=w329:bool)
          n115 = Bundle By Name(cluster=T4 {"Row"=0, "Column"=0} ("Active Cell:Active Cell"), "Row"=w309, "Column"=1) -> (w301:T4)
          n116 = Select(t=u32 65280 ("Active Cell:Cell Background Color"), s=w327, f=u32 16711680 ("Active Cell:Cell Background Color")) -> (s? t:f=w298:u32)
          n117 = property class="MCListbox (strict)"(reference=w323, "ActiveCell"=w301) -> (reference out=w322:refnum<vi>)  [unwired: 1 in, 1 out]
          n118 = property class="MCListbox (strict)"(reference=w322, "CellBG"=w298) -> (reference out=w302:refnum<vi>)  [unwired: 1 in, 1 out]
          n119 = Bundle By Name(cluster=w301, "Column"=2) -> (w299:T4)
          n120 = Greater?(x=w309, y=1) -> (0:w307:bool)
          n121 = property class="MCListbox (strict)"(reference=w302, "ActiveCell"=w299) -> (reference out=w303:refnum<vi>)  [unwired: 1 in, 1 out]
          n122 = property class="MCListbox (strict)"(reference=w303, "CellBG"=w298) -> ()  [unwired: 1 in, 2 out]
          n123 = Number To Fractional String(number=w311, precision (6)=w310) -> (F-format string=w306:string)  [unwired: 2 out]
          n124 = Select(t="NA", s=w307, f=w306) -> (s? t:f=w304:string)
          n125 = Number To Fractional String(number=w332, precision (6)=w310) -> (F-format string=w321:string)  [unwired: 2 out]
        }
        n126 = property class="MCListbox (strict)"(reference=w288) -> (reference out=w292:refnum<vi>, "ItemNames"=w291:string[][])  [unwired: 1 in, 1 out]
        n127 = Replace Array Subset(array=w291, new element=w289, index (col)=1 ("disabled index (col)")) -> (w284:string[][])  [unwired: 1 in]
        n128 = Replace Array Subset(array=w284, new element=w281, index (col)=2 ("disabled index (col)")) -> (w283:string[][])  [unwired: 1 in]
        n129 = property class="MCListbox (strict)"(reference=w292, "ItemNames"=w283) -> ()  [unwired: 1 in, 2 out]
      }
      frame #5 {
        w336 = u8[] [90, 91, 91, 91, 91]  # ADC I Ch#
        w349 = u8[] [88, 89, 92, 93, 94]  # ADC V Ch#
        n130 = for {
          tunnel: w349 -> [w368] mode=indexing
          tunnel: dbl[] [420.0, -420.0, 5.0, -5.0, 2.3] ("VoltageInput 2") -> [w383] mode=indexing
          tunnel: w347 -> [w366]
          tunnel: w346 -> [w364]
          shift-right: [w381] -> w333
          shift-left: TRUE -> [w382]
          tunnel: w334 -> [w375]
          tunnel: [w373] -> w341 mode=indexing
          tunnel: w340 -> [w365]
          tunnel: w336 -> [w367] mode=indexing
          tunnel: [w356] -> w335 mode=indexing
          i -> [w361]
          w362 = i16 3 ("precision (6)")
          n131 = call "_Remote Calculate ADC.vi"("ADC Table"=w364, "Unit"=w365, "ADC Channel (64)"=w368, "ADC Values"=w366) -> ("User Value"=w384:dbl)  [unwired: 3 out]
          n132 = call "_Remote Calculate ADC.vi"("ADC Table"=w364, "Unit"=w365, "ADC Channel (64)"=w367, "ADC Values"=w366) -> ("User Value"=w363:dbl)  [unwired: 3 out]
          n133 = Index Array(array=w364, index=w368) -> (element=w370:T3)
          n134 = Unbundle By Name(w370) -> ("Min"=w369:dbl)
          n135 = Add(x=w383, y=w369) -> (x+y=w372:dbl)
          n136 = Subtract(x=w383, y=w369) -> (x-y=w371:dbl)
          n137 = In Range and Coerce(upper limit=w372, x=w384, lower limit=w371) -> (In Range?=w379:bool)  [unwired: 1 out]
          n138 = And(x=w379, y=w382) -> (x .and. y?=w381:bool)
          n139 = Bundle By Name(cluster=T4 {"Row"=0, "Column"=0} ("Active Cell:Active Cell"), "Row"=w361, "Column"=1) -> (w353:T4)
          n140 = Select(t=u32 65280 ("Active Cell:Cell Background Color"), s=w379, f=u32 16711680 ("Active Cell:Cell Background Color")) -> (s? t:f=w350:u32)
          n141 = property class="MCListbox (strict)"(reference=w375, "ActiveCell"=w353) -> (reference out=w374:refnum<vi>)  [unwired: 1 in, 1 out]
          n142 = property class="MCListbox (strict)"(reference=w374, "CellBG"=w350) -> (reference out=w354:refnum<vi>)  [unwired: 1 in, 1 out]
          n143 = Bundle By Name(cluster=w353, "Column"=2) -> (w351:T4)
          n144 = Greater?(x=w361, y=1) -> (0:w359:bool)
          n145 = property class="MCListbox (strict)"(reference=w354, "ActiveCell"=w351) -> (reference out=w355:refnum<vi>)  [unwired: 1 in, 1 out]
          n146 = property class="MCListbox (strict)"(reference=w355, "CellBG"=w350) -> ()  [unwired: 1 in, 2 out]
          n147 = Number To Fractional String(number=w384, precision (6)=w362) -> (F-format string=w373:string)  [unwired: 2 out]
          n148 = Number To Fractional String(number=w363, precision (6)=w362) -> (F-format string=w358:string)  [unwired: 2 out]
          n149 = Select(t="NA", s=w359, f=w358) -> (s? t:f=w356:string)
        }
        n150 = property class="MCListbox (strict)"(reference=w334) -> (reference out=w344:refnum<vi>, "ItemNames"=w343:string[][])  [unwired: 1 in, 1 out]
        n151 = Replace Array Subset(array=w343, new element=w341, index (col)=1 ("disabled index (col)")) -> (w338:string[][])  [unwired: 1 in]
        n152 = Replace Array Subset(array=w338, new element=w335, index (col)=2 ("disabled index (col)")) -> (w337:string[][])  [unwired: 1 in]
        n153 = property class="MCListbox (strict)"(reference=w344, "ItemNames"=w337) -> ()  [unwired: 1 in, 2 out]
      }
      frame #6 {
        w389 = u8[] [22, 23]  # ADC I Ch#
        w401 = u8[] [20, 21]  # ADC V Ch#
        n154 = for {
          tunnel: w401 -> [w415] mode=indexing
          tunnel: dbl[] [600.0, -600.0] ("VoltageInput 2") -> [w431] mode=indexing
          tunnel: w399 -> [w412]
          tunnel: w398 -> [w411]
          shift-right: [w429] -> w391
          shift-left: TRUE -> [w430]
          tunnel: w392 -> [w422]
          tunnel: [w420] -> w393 mode=indexing
          tunnel: w390 -> [w413]
          tunnel: w389 -> [w414] mode=indexing
          tunnel: [w409] -> w385 mode=indexing
          i -> [w423]
          w402 = i16 3 ("precision (6)")
          n155 = call "_Remote Calculate ADC.vi"("ADC Table"=w411, "Unit"=w413, "ADC Channel (64)"=w415, "ADC Values"=w412) -> ("User Value"=w432:dbl)  [unwired: 3 out]
          n156 = call "_Remote Calculate ADC.vi"("ADC Table"=w411, "Unit"=w413, "ADC Channel (64)"=w414, "ADC Values"=w412) -> ("User Value"=w410:dbl)  [unwired: 3 out]
          n157 = Index Array(array=w411, index=w415) -> (element=w417:T3)
          n158 = Unbundle By Name(w417) -> ("Min"=w416:dbl)
          n159 = Add(x=w431, y=w416) -> (x+y=w419:dbl)
          n160 = Subtract(x=w431, y=w416) -> (x-y=w418:dbl)
          n161 = In Range and Coerce(upper limit=w419, x=w432, lower limit=w418) -> (In Range?=w427:bool)  [unwired: 1 out]
          n162 = And(x=w427, y=w430) -> (x .and. y?=w429:bool)
          n163 = Bundle By Name(cluster=T4 {"Row"=0, "Column"=0} ("Active Cell:Active Cell"), "Row"=w423, "Column"=1) -> (w405:T4)
          n164 = Select(t=u32 65280 ("Active Cell:Cell Background Color"), s=w427, f=u32 16711680 ("Active Cell:Cell Background Color")) -> (s? t:f=w406:u32)
          n165 = property class="MCListbox (strict)"(reference=w422, "ActiveCell"=w405) -> (reference out=w421:refnum<vi>)  [unwired: 1 in, 1 out]
          n166 = property class="MCListbox (strict)"(reference=w421, "CellBG"=w406) -> (reference out=w407:refnum<vi>)  [unwired: 1 in, 1 out]
          n167 = Bundle By Name(cluster=w405, "Column"=2) -> (w403:T4)
          n168 = property class="MCListbox (strict)"(reference=w407, "ActiveCell"=w403) -> (reference out=w408:refnum<vi>)  [unwired: 1 in, 1 out]
          n169 = property class="MCListbox (strict)"(reference=w408, "CellBG"=w406) -> ()  [unwired: 1 in, 2 out]
          n170 = Number To Fractional String(number=w432, precision (6)=w402) -> (F-format string=w420:string)  [unwired: 2 out]
          n171 = Number To Fractional String(number=w410, precision (6)=w402) -> (F-format string=w409:string)  [unwired: 2 out]
        }
        n172 = property class="MCListbox (strict)"(reference=w392) -> (reference out=w396:refnum<vi>, "ItemNames"=w395:string[][])  [unwired: 1 in, 1 out]
        n173 = Replace Array Subset(array=w395, new element=w393, index (col)=1 ("disabled index (col)")) -> (w387:string[][])  [unwired: 1 in]
        n174 = Replace Array Subset(array=w387, new element=w385, index (col)=2 ("disabled index (col)")) -> (w386:string[][])  [unwired: 1 in]
        n175 = property class="MCListbox (strict)"(reference=w396, "ItemNames"=w386) -> ()  [unwired: 1 in, 2 out]
      }
      frame #7 {
        w444 = 1 ("disabled index (col)")
        w454 = "Not Used"
        w465 = u8[] [64, 65, 67, 66, 68, 71]  # ADC Ch#
        # "need to take out the 70"
        n176 = call "_Remote Calculate ADC.vi"("ADC Channel (64)"=u8 113, "ADC Values"=w436) -> ("Raw Reading"=w438:dbl)  [unwired: 2 in, 3 out]
        n177 = call "_Remote Calculate ADC.vi"("ADC Channel (64)"=u8 114, "ADC Values"=w436) -> ("Raw Reading"=w437:dbl)  [unwired: 2 in, 3 out]
        n178 = To Byte Integer(number=w437) -> (8bit integer=w434:i8)
        n179 = To Byte Integer(number=w438) -> (8bit integer=w435:i8)
        n180 = for {
          tunnel: w465 -> [w472] mode=indexing
          tunnel: w436 -> [w503]
          tunnel: w464 -> [w489]
          shift-right: [w501] -> w458
          shift-left: TRUE -> [w502]
          tunnel: w459 -> [w495]
          tunnel: [w492] -> w460 mode=indexing
          tunnel: w457 -> [w490]
          tunnel: w456 -> [w481] mode=indexing
          tunnel: w455 -> [w486]
          tunnel: [w480] -> w443 mode=indexing
          tunnel: w442 -> [w483]
          tunnel: w441 -> [w482]
          tunnel: w435 -> [w479]
          tunnel: w434 -> [w478]
          i -> [w496]
          w477 = i8 4 ("y")
          n181 = Greater Than 0?(x=w481) -> (x > 0?=w480:bool)
          n182 = Equal?(x=u8 66, y=w472) -> (x = y?=w475:bool)
          n183 = Equal?(x=u8 67, y=w472) -> (x = y?=w471:bool)
          n184 = Equal?(x=w472, y=u8 68) -> (x = y?=w470:bool)
          n185 = Or(x=w475, y=w470) -> (x .or. y?=w485:bool)
          n186 = Equal?(x=w479, y=w477) -> (x = y?=w474:bool)
          n187 = Equal?(x=w477, y=w478) -> (x = y?=w476:bool)
          n188 = Bundle By Name(cluster=T4 {"Row"=0, "Column"=0} ("Active Cell:Active Cell"), "Row"=w496, "Column"=3) -> (w491:T4)
          n189 = property class="Tbl (strict)"(reference=w495, "Active Cell"=w491) -> (reference out=w494:refnum<vi>)  [unwired: 1 in, 1 out]
          n190 = And(x=w486, y=w485) -> (x .and. y?=w469:bool)
          n191 = And(x=w474, y=w471) -> (x .and. y?=w468:bool)
          n192 = And(x=w476, y=w470) -> (x .and. y?=w467:bool)
          n193 = Compound Arithmetic op=OR(w469, w468, w467) -> (w466:bool)
          n194 = case shown="False" w466 {
            tunnel: w503 -> [w525 _]
            tunnel: [w509 "NA"] -> w492
            tunnel: w490 -> [w523 _]
            tunnel: w489 -> [w518 _]
            tunnel: w481 -> [w517 _]
            tunnel: [w505 TRUE] -> w484
            tunnel: w472 -> [w515 _]
            frame False {
              n195 = call "_Remote Calculate ADC.vi"("ADC Table"=w518, "Unit"=w523, "ADC Channel (64)"=w515, "ADC Values"=w525) -> ("User Value"=w504:dbl)  [unwired: 3 out]
              n196 = Index Array(array=w518, index=w515) -> (element=w520:T3)
              n197 = Unbundle By Name(w520) -> ("Min"=w519:dbl)
              n198 = Less?(x=w504, y=1.0) -> (x < y?=w506:bool)
              n199 = Add(x=w517, y=w519) -> (x+y=w522:dbl)
              n200 = Subtract(x=w517, y=w519) -> (x-y=w521:dbl)
              n201 = Select(t="ON", s=w506, f="OFF" ("t")) -> (s? t:f=w511:string)
              n202 = In Range and Coerce(upper limit=w522, x=w504, lower limit=w521) -> (In Range?=w507:bool)  [unwired: 1 out]
              n203 = Number To Fractional String(number=w504, precision (6)=i16 3) -> (F-format string=w510:string)  [unwired: 2 out]
              n204 = Equal?(x=u8 70, y=w515) -> (x = y?=w508:bool)
              n205 = Select(t=w506, s=w508, f=w507) -> (s? t:f=w505:bool)
              n206 = Select(t=w511, s=w508, f=w510) -> (s? t:f=w509:string)
            }
            frame True {
              # "In cases:\n1. if Single Source, NG2 = NA;\n2. if Single Source, HG2 = NA;\n3. if S1=MicroSpray, HG1 = NA;\n4. if S2=MicroSpray, HG2 = NA."
            }
          }
          n207 = call "_Update Ion Path.vi"("Value"=w481, "Source Map"=w483, "Voltage OK"=w484, "ADC Ch#"=w472, "Ion Path"=w482) -> ()  [unwired: 2 in, 3 out]
          n208 = And(x=w484, y=w502) -> (x .and. y?=w501:bool)
          n209 = Select(t=u32 65280 ("Active Cell:Cell Background Color"), s=w484, f=u32 16711680 ("Active Cell:Cell Background Color")) -> (s? t:f=w493:u32)
          n210 = property class="Tbl (strict)"(reference=w494, "Cell BG Color"=w493) -> ()  [unwired: 1 in, 2 out]
        }
        n211 = Select(t=w454, s=w455, f="NG2") -> (s? t:f=w446:string)
        n212 = Select(t=w454, s=w455, f="HG2") -> (s? t:f=w445:string)
        n213 = property class="Tbl (strict)"(reference=w459) -> (reference out=w462:refnum<vi>, "Value"=w451:string[][])  [unwired: 1 in, 1 out]
        n214 = Replace Array Subset(array=w451, new element=w446, index (row)=3 ("disabled index (col)"), index (col)=w444) -> (w450:string[][])
        n215 = Replace Array Subset(array=w450, new element=w445, index (row)=4 ("disabled index (col)"), index (col)=w444) -> (w449:string[][])
        n216 = Replace Array Subset(array=w449, new element=w460, index (col)=3 ("disabled index (col)")) -> (w433:string[][])  [unwired: 1 in]
        n217 = property class="Tbl (strict)"(reference=w462, "Value"=w433) -> ()  [unwired: 1 in, 2 out]
      }
      frame #8 {
        w556 = u8[] [105, 110, 108]  # ADC Ch#
        n218 = Index Array(array=w536, index #1=0 ("index"), index #2=2 ("index"), index #3=4 ("index")) -> (element #1=w530:dbl, element #2=w531:dbl, element #3=w532:dbl)
        n219 = Build Array(w530, w531, w532) -> (w529:dbl[])
        n220 = for {
          tunnel: w556 -> [w570] mode=indexing
          tunnel: w555 -> [w585]
          tunnel: w554 -> [w572]
          shift-right: [w584] -> w547
          shift-left: TRUE -> [w571]
          tunnel: w548 -> [w578]
          tunnel: [w575] -> w550 mode=indexing
          tunnel: w546 -> [w573]
          tunnel: w545 -> [w558] mode=indexing
          tunnel: w538 -> [w568]
          tunnel: w529 -> [w563] mode=indexing
          tunnel: [w557] -> w528 mode=indexing
          i -> [w579]
          n221 = Greater Than 0?(x=w558) -> (x > 0?=w557:bool)
          n222 = Less?(x=w558, y=75.0) -> (x < y?=w561:bool)
          n223 = Less?(x=w563, y=225.0) -> (x < y?=w562:bool)
          n224 = Equal?(x=u8 108, y=w570) -> (x = y?=w567:bool)
          n225 = Or(x=w562, y=w561) -> (x .or. y?=w560:bool)
          n226 = And(x=w568, y=w567) -> (x .and. y?=w566:bool)
          n227 = Bundle By Name(cluster=T4 {"Row"=0, "Column"=0} ("Active Cell:Active Cell"), "Row"=w579, "Column"=3) -> (w574:T4)
          n228 = property class="Tbl (strict)"(reference=w578, "Active Cell"=w574) -> (reference out=w577:refnum<vi>)  [unwired: 1 in, 1 out]
          n229 = case shown="False" w566 {
            tunnel: w585 -> [w596 _]
            tunnel: [w595 "NA"] -> w575
            tunnel: w573 -> [w594 _]
            tunnel: w572 -> [w593 _]
            tunnel: [w592 TRUE] -> w559
            tunnel: w558 -> [w590 _]
            tunnel: w570 -> [w587 _]
            tunnel: w560 -> [w586 _]
            frame False {
              n230 = Not Equal?(x=w587, y=u8 105) -> (x != y?=w589:bool)
              n231 = And(x=w589, y=w586) -> (x .and. y?=w588:bool)
              n232 = case shown="False" w588 {
                tunnel: w596 -> [w609 _]
                tunnel: [w607 "OFF"] -> w595
                tunnel: w594 -> [w606 _]
                tunnel: w593 -> [w601 _]
                tunnel: [w599 TRUE] -> w592
                tunnel: w587 -> [w598 _]
                tunnel: w590 -> [w597 _]
                frame False {
                  n233 = call "_Remote Calculate ADC.vi"("ADC Table"=w601, "Unit"=w606, "ADC Channel (64)"=w598, "ADC Values"=w609) -> ("User Value"=w600:dbl)  [unwired: 3 out]
                  n234 = Index Array(array=w601, index=w598) -> (element=w603:T3)
                  n235 = Unbundle By Name(w603) -> ("Min"=w602:dbl)
                  n236 = Add(x=w597, y=w602) -> (x+y=w605:dbl)
                  n237 = Subtract(x=w597, y=w602) -> (x-y=w604:dbl)
                  n238 = In Range and Coerce(upper limit=w605, x=w600, lower limit=w604) -> (In Range?=w599:bool)  [unwired: 1 out]
                  n239 = Number To Fractional String(number=w600, precision (6)=i16 3) -> (F-format string=w607:string)  [unwired: 2 out]
                }
                frame True {
                  # "Prob temp reports OFF if\nHG is set to < 225\nor PT is set to < 75"
                }
              }
            }
            frame True {
            }
          }
          n240 = And(x=w559, y=w571) -> (x .and. y?=w584:bool)
          n241 = Select(t=u32 65280 ("Active Cell:Cell Background Color"), s=w559, f=u32 16711680 ("Active Cell:Cell Background Color")) -> (s? t:f=w576:u32)
          n242 = property class="Tbl (strict)"(reference=w577, "Cell BG Color"=w576) -> ()  [unwired: 1 in, 2 out]
        }
        n243 = Select(t="Not Used", s=w538, f="P2T") -> (s? t:f=w537:string)
        n244 = property class="Tbl (strict)"(reference=w548) -> (reference out=w552:refnum<vi>, "Value"=w542:string[][])  [unwired: 1 in, 1 out]
        n245 = Replace Array Subset(array=w542, new element=w537, index (row)=2 ("disabled index (col)"), index (col)=1 ("disabled index (col)")) -> (w541:string[][])
        n246 = Replace Array Subset(array=w541, new element=w550, index (col)=3 ("disabled index (col)")) -> (w549:string[][])  [unwired: 1 in]
        n247 = property class="Tbl (strict)"(reference=w552, "Value"=w549) -> ()  [unwired: 1 in, 2 out]
      }
      frame #9 {
        w647 = u8[] [107, 109]  # ADC Ch#
        n248 = call "_Remote Calculate ADC.vi"("ADC Channel (64)"=u8 113, "ADC Values"=w638) -> ("Raw Reading"=w630:dbl)  [unwired: 2 in, 3 out]
        n249 = call "_Remote Calculate ADC.vi"("ADC Channel (64)"=u8 114, "ADC Values"=w638) -> ("Raw Reading"=w629:dbl)  [unwired: 2 in, 3 out]
        n250 = To Byte Integer(number=w629) -> (8bit integer=w625:i8)
        n251 = To Byte Integer(number=w630) -> (8bit integer=w637:i8)
        "Source 1 Type:" <- w637
        n252 = Select(t=i8 0, s=w615, f=w625) -> (s? t:f=w623:i8)
        "Source 2 Type:" <- w623
        n253 = case shown="4" w637 {
          tunnel: ["None" "ESI" "APCI" "APPI" "MicroSpray"] -> w636
          frame 0, Default {
          }
          frame 1 {
          }
          frame 2 {
          }
          frame 3 {
          }
          frame 4 {
          }
        }
        n254 = case shown="4" w623 {
          tunnel: ["None" "ESI" "APCI" "APPI" "MicroSpray"] -> w635
          frame 0, Default {
          }
          frame 1 {
          }
          frame 2 {
          }
          frame 3 {
          }
          frame 4 {
          }
        }
        n255 = for {
          tunnel: w647 -> [w659] mode=indexing
          tunnel: w638 -> [w680]
          tunnel: w646 -> [w666]
          shift-right: [w678] -> w641
          shift-left: TRUE -> [w679]
          tunnel: w642 -> [w674]
          tunnel: [w671] -> w628 mode=indexing
          tunnel: w631 -> [w669]
          tunnel: w626 -> [w664] mode=indexing
          tunnel: w615 -> [w663]
          tunnel: w614 -> [w658]
          i -> [w667]
          n256 = Equal?(x=u8 109, y=w659) -> (x = y?=w662:bool)
          n257 = And(x=w663, y=w662) -> (x .and. y?=w661:bool)
          n258 = Bundle By Name(cluster=T4 {"Row"=0, "Column"=0} ("Active Cell:Active Cell"), "Row"=w667, "Column"=3) -> (w670:T4)
          n259 = case shown="False" w661 {
            tunnel: w680 -> [w696 _]
            tunnel: [w694 "NA"] -> w671
            tunnel: w669 -> [w693 _]
            tunnel: w666 -> [w688 _]
            tunnel: [w687 TRUE] -> w660
            tunnel: w659 -> [w683 _]
            tunnel: w664 -> [w682 _]
            frame False {
              n260 = call "_Remote Calculate ADC.vi"("ADC Table"=w688, "Unit"=w693, "ADC Channel (64)"=w683, "ADC Values"=w696) -> ("User Value"=w685:dbl)  [unwired: 3 out]
              n261 = Index Array(array=w688, index=w683) -> (element=w690:T3)
              n262 = Unbundle By Name(w690) -> ("Min"=w689:dbl)
              n263 = Greater Or Equal To 0?(x=w682) -> (x >= 0?=w686:bool)
              n264 = Negate(x=w685) -> (-x=w684:dbl)
              n265 = Add(x=w682, y=w689) -> (x+y=w692:dbl)
              n266 = Subtract(x=w682, y=w689) -> (x-y=w691:dbl)
              n267 = Select(t=w685, s=w686, f=w684) -> (s? t:f=w681:dbl)
              n268 = In Range and Coerce(upper limit=w692, x=w681, lower limit=w691) -> (In Range?=w687:bool)  [unwired: 1 out]
              n269 = Number To Fractional String(number=w681, precision (6)=i16 3) -> (F-format string=w694:string)  [unwired: 2 out]
            }
            frame True {
            }
          }
          n270 = property class="Tbl (strict)"(reference=w674, "Active Cell"=w670) -> (reference out=w673:refnum<vi>)  [unwired: 1 in, 1 out]
          n271 = call "_Update Ion Path.vi"("Source Map"=w658, "Voltage OK"=w660, "ADC Ch#"=w659) -> ()  [unwired: 4 in, 3 out]
          n272 = And(x=w660, y=w679) -> (x .and. y?=w678:bool)
          n273 = Select(t=u32 65280 ("Active Cell:Cell Background Color"), s=w660, f=u32 16711680 ("Active Cell:Cell Background Color")) -> (s? t:f=w672:u32)
          n274 = property class="Tbl (strict)"(reference=w673, "Cell BG Color"=w672) -> ()  [unwired: 1 in, 2 out]
        }
        n275 = property class="Tbl (strict)"(reference=w642) -> (reference out=w644:refnum<vi>, "Value"=w620:string[][])  [unwired: 1 in, 1 out]
        n276 = Select(t="Not Used", s=w615, f="Pillar 2") -> (s? t:f=w616:string)
        n277 = Replace Array Subset(array=w620, new element=w616, index (row)=1 ("disabled index (col)"), index (col)=0 ("disabled index (col)")) -> (w619:string[][])
        n278 = Build Array(w636, w635) -> (w632:string[])
        n279 = Replace Array Subset(array=w619, new element=w632, index (col)=1 ("disabled index (col)")) -> (w633:string[][])  [unwired: 1 in]
        n280 = Replace Array Subset(array=w633, new element=w628, index (col)=3 ("disabled index (col)")) -> (w627:string[][])  [unwired: 1 in]
        n281 = property class="Tbl (strict)"(reference=w644, "Value"=w627) -> ()  [unwired: 1 in, 2 out]
      }
      frame #10 {
        w701 = u8[] [106, 104]  # ADC Ch#
        n282 = for {
          tunnel: w701 -> [w718] mode=indexing
          tunnel: w713 -> [w744]
          tunnel: w712 -> [w727]
          shift-right: [w741] -> w706
          shift-left: TRUE -> [w742]
          tunnel: w707 -> [w719]
          tunnel: [w735] -> w704 mode=indexing
          tunnel: w705 -> [w734]
          tunnel: w702 -> [w724] mode=indexing
          tunnel: w700 -> [w721]
          tunnel: w699 -> [w714]
          i -> [w732]
          n283 = call "_Remote Calculate ADC.vi"("ADC Table"=w727, "Unit"=w734, "ADC Channel (64)"=w718, "ADC Values"=w744) -> ("User Value"=w725:dbl)  [unwired: 3 out]
          n284 = Index Array(array=w727, index=w718) -> (element=w729:T3)
          n285 = Greater Or Equal To 0?(x=w724) -> (x >= 0?=w723:bool)
          n286 = Unbundle By Name(w729) -> ("Min"=w728:dbl)
          n287 = Negate(x=w725) -> (-x=w726:dbl)
          n288 = Add(x=w724, y=w728) -> (x+y=w731:dbl)
          n289 = Subtract(x=w724, y=w728) -> (x-y=w730:dbl)
          n290 = Select(t=w725, s=w723, f=w726) -> (s? t:f=w722:dbl)
          n291 = Bundle By Name(cluster=T4 {"Row"=0, "Column"=0} ("Active Cell:Active Cell"), "Row"=w732, "Column"=2) -> (w716:T4)
          n292 = property class="Tbl (strict)"(reference=w719, "Active Cell"=w716) -> (reference out=w737:refnum<vi>)  [unwired: 1 in, 1 out]
          n293 = Bundle By Name(cluster=w716, "Column"=1 ("Row")) -> (w715:T4)
          n294 = In Range and Coerce(upper limit=w731, x=w722, lower limit=w730) -> (In Range?=w720:bool)  [unwired: 1 out]
          n295 = call "_Update Ion Path.vi"("Source Map"=w714, "Current Cell"=w715, "Voltage OK"=w720, "ADC Ch#"=w718, "Lens Table"=w719, "Ion Path"=w721) -> ()  [unwired: 1 in, 3 out]
          n296 = And(x=w720, y=w742) -> (x .and. y?=w741:bool)
          n297 = Select(t=u32 65280 ("Active Cell:Cell Background Color"), s=w720, f=u32 16711680 ("Active Cell:Cell Background Color")) -> (s? t:f=w736:u32)
          n298 = property class="Tbl (strict)"(reference=w737, "Cell BG Color"=w736) -> ()  [unwired: 1 in, 2 out]
          n299 = Number To Fractional String(number=w722, precision (6)=i16 3) -> (F-format string=w735:string)  [unwired: 2 out]
        }
        n300 = property class="Tbl (strict)"(reference=w707) -> (reference out=w710:refnum<vi>, "Value"=w709:string[][])  [unwired: 1 in, 1 out]
        n301 = Replace Array Subset(array=w709, new element=w704, index (col)=2 ("disabled index (col)")) -> (w703:string[][])  [unwired: 1 in]
        n302 = property class="Tbl (strict)"(reference=w710, "Value"=w703) -> ()  [unwired: 1 in, 2 out]
      }
      frame #11 {
        w766 = u8[] [74, 119, 72, 76, 78]  # ADC Ch#
        n303 = for {
          tunnel: w766 -> [w778] mode=indexing
          tunnel: w765 -> [w795]
          tunnel: w764 -> [w794]
          shift-right: [w792] -> w761
          shift-left: TRUE -> [w793]
          tunnel: w760 -> [w786]
          tunnel: [w780] -> w749 mode=indexing
          tunnel: w757 -> [w781]
          shift-right: [w775] -> w755
          shift-left: w754 -> [w773]
          shift-right: [w774] -> w753
          shift-left: w752 -> [w771]
          tunnel: w751 -> [w772]
          tunnel: w750 -> [w770]
          tunnel: w747 -> [w769]
          i -> [w787]
          n304 = case shown="76, 78" w778 {
            tunnel: ["%.2f" ("format string") "%.2e" ("format string") "%.2g" ("format string")] -> w779
            frame 0, Default {
            }
            frame 119 {
            }
            frame 76, 78 {
            }
          }
          n305 = call "_Remote Calculate ADC.vi"("ADC Table"=w794, "Unit"=w781, "ADC Channel (64)"=w778, "ADC Values"=w795) -> ("In Range?"=w782:bool, "User Value"=w777:dbl)  [unwired: 2 out]
          n306 = Less Or Equal?(x=w769, y=u32 2) -> (x <= y?=w767:bool)
          n307 = case shown="74" w778 {
            tunnel: w777 -> [w798 w800 w810]
            tunnel: [w798 w799 w808] -> w776
            tunnel: [w797 w800 w816] -> w775
            tunnel: [w796 w807 w810] -> w774
            tunnel: w773 -> [w797 w804 w816]
            tunnel: w772 -> [_ w803 _]
            tunnel: w771 -> [w796 w807 w815]
            tunnel: w770 -> [_ _ w814]
            tunnel: w767 -> [_ w802 w811]
            frame 0, Default {
            }
            frame 74 {
              n308 = Compound Arithmetic op=ADD(w800, w804, w803) -> (w806:dbl)
              n309 = Divide(x=w806, y=3.0) -> (x/y=w801:dbl)
              n310 = Select(t=w800, s=w802, f=w801) -> (s? t:f=w799:dbl)
            }
            frame 72 {
              n311 = Compound Arithmetic op=ADD(w810, w815, w814) -> (w813:dbl)
              n312 = Divide(x=w813, y=3.0) -> (x/y=w809:dbl)
              n313 = Select(t=w810, s=w811, f=w809) -> (s? t:f=w808:dbl)
            }
          }
          n314 = And(x=w782, y=w793) -> (x .and. y?=w792:bool)
          n315 = Bundle By Name(cluster=T4 {"Row"=0, "Column"=0} ("Active Cell:Active Cell"), "Row"=w787, "Column"=1) -> (w783:T4)
          n316 = property class="Tbl (strict)"(reference=w786, "Active Cell"=w783) -> (reference out=w785:refnum<vi>)  [unwired: 1 in, 1 out]
          n317 = Select(t=u32 65280 ("Active Cell:Cell Background Color"), s=w782, f=u32 16711680 ("Active Cell:Cell Background Color")) -> (s? t:f=w784:u32)
          n318 = property class="Tbl (strict)"(reference=w785, "Cell BG Color"=w784) -> ()  [unwired: 1 in, 2 out]
          n319 = Format Into String(format string=w779, w776) -> (resulting string=w780:string)  [unwired: 2 in, 1 out]
        }
        n320 = Select(t=string[][] [["Foreline Pressure (Pa)", "0"], ["Analyzer Pressure (Pa)", "0"], ["Plenum Delta P (Pa)", ""], ["Drying Gas Pressure (Pa)", ""], ["Source Gas Pressure (Pa)", ""]] ("Vacuum Readings by Region"), s=w757, f=string[][] [["Foreline Pressure (torr)", "0"], ["Analyzer Pressure (torr)", "0"], ["Plenum Delta P (torr)", ""], ["Drying Gas Pressure (psi)", ""], ["Source Gas Pressure (psi)", ""]] ("Vacuum Readings by Region")) -> (s? t:f=w756:string[][])
        n321 = Replace Array Subset(array=w756, new element=w749, index (col)=1 ("disabled index (col)")) -> (w746:string[][])  [unwired: 1 in]
        n322 = property class="Tbl (strict)"(reference=w760, "Value"=w746) -> ()  [unwired: 1 in, 2 out]
        n323 = Array Subset(array=w746, length (row)=2 ("length")) -> (→"Pressure":string[][])  [unwired: 3 in]
      }
      frame #12 {
        w831 = u8[] [16, 17, 18, 19]  # ADC Ch#
        n324 = for {
          tunnel: w831 -> [w847] mode=indexing
          tunnel: w830 -> [w848]
          tunnel: w829 -> [w846]
          shift-right: [w832] -> w824
          shift-left: TRUE -> [w832]
          tunnel: w821 -> [w838]
          tunnel: [w835] -> w826 mode=indexing
          tunnel: w823 -> [w833]
          i -> [w839]
          n325 = call "_Remote Calculate ADC.vi"("ADC Table"=w846, "Unit"=w833, "ADC Channel (64)"=w847, "ADC Values"=w848) -> ("User Value"=w844:dbl)  [unwired: 3 out]
          n326 = Bundle By Name(cluster=T4 {"Row"=0, "Column"=0} ("Active Cell:Active Cell"), "Row"=w839, "Column"=1) -> (w834:T4)
          n327 = Select(t=u32 65280 ("Active Cell:Cell Background Color"), s=w832, f=u32 16711680 ("Active Cell:Cell Background Color")) -> (s? t:f=w836:u32)
          n328 = property class="Tbl (strict)"(reference=w838, "Active Cell"=w834) -> (reference out=w837:refnum<vi>)  [unwired: 1 in, 1 out]
          n329 = property class="Tbl (strict)"(reference=w837, "Cell BG Color"=w836) -> ()  [unwired: 1 in, 2 out]
          n330 = Number To Fractional String(number=w844, precision (6)=i16 3) -> (F-format string=w835:string)  [unwired: 2 out]
        }
        n331 = property class="Tbl (strict)"(reference=w821) -> (reference out=w822:refnum<vi>, "Value"=w820:string[][])  [unwired: 1 in, 1 out]
        n332 = Replace Array Subset(array=w820, new element=w826, index (col)=1 ("disabled index (col)")) -> (w825:string[][])  [unwired: 1 in]
        n333 = property class="Tbl (strict)"(reference=w822, "Value"=w825) -> ()  [unwired: 1 in, 2 out]
      }
      frame #13 {
        w860 = u8[] [57, 58]  # ADC Ch#
        n334 = for {
          tunnel: w860 -> [w878] mode=indexing
          tunnel: w859 -> [w879]
          tunnel: w858 -> [w877]
          shift-right: [w862] -> w849
          shift-left: TRUE -> [w863]
          tunnel: w850 -> [w869]
          tunnel: [w866] -> w855 mode=indexing
          tunnel: w853 -> [w864]
          i -> [w870]
          n335 = call "_Remote Calculate ADC.vi"("ADC Table"=w877, "Unit"=w864, "ADC Channel (64)"=w878, "ADC Values"=w879) -> ("In Range?"=w861:bool, "User Value"=w875:dbl)  [unwired: 2 out]
          n336 = And(x=w861, y=w863) -> (x .and. y?=w862:bool)
          n337 = Bundle By Name(cluster=T4 {"Row"=0, "Column"=0} ("Active Cell:Active Cell"), "Row"=w870, "Column"=1) -> (w865:T4)
          n338 = property class="Tbl (strict)"(reference=w869, "Active Cell"=w865) -> (reference out=w868:refnum<vi>)  [unwired: 1 in, 1 out]
          n339 = Select(t=u32 65280 ("Active Cell:Cell Background Color"), s=w861, f=u32 16711680 ("Active Cell:Cell Background Color")) -> (s? t:f=w867:u32)
          n340 = property class="Tbl (strict)"(reference=w868, "Cell BG Color"=w867) -> ()  [unwired: 1 in, 2 out]
          n341 = Number To Fractional String(number=w875, precision (6)=i16 3) -> (F-format string=w866:string)  [unwired: 2 out]
        }
        n342 = property class="Tbl (strict)"(reference=w850) -> (reference out=w852:refnum<vi>, "Value"=w851:string[][])  [unwired: 1 in, 1 out]
        n343 = Replace Array Subset(array=w851, new element=w855, index (col)=1 ("disabled index (col)")) -> (w854:string[][])  [unwired: 1 in]
        n344 = property class="Tbl (strict)"(reference=w852, "Value"=w854) -> ()  [unwired: 1 in, 2 out]
      }
      frame #14 {
        w891 = u8[] [49, 50]  # ADC Ch#
        n345 = for {
          tunnel: w891 -> [w909] mode=indexing
          tunnel: w890 -> [w910]
          tunnel: w889 -> [w908]
          shift-right: [w893] -> w880
          shift-left: TRUE -> [w894]
          tunnel: w881 -> [w900]
          tunnel: [w897] -> w886 mode=indexing
          tunnel: w884 -> [w895]
          i -> [w901]
          n346 = call "_Remote Calculate ADC.vi"("ADC Table"=w908, "Unit"=w895, "ADC Channel (64)"=w909, "ADC Values"=w910) -> ("In Range?"=w892:bool, "User Value"=w906:dbl)  [unwired: 2 out]
          n347 = And(x=w892, y=w894) -> (x .and. y?=w893:bool)
          n348 = Bundle By Name(cluster=T4 {"Row"=0, "Column"=0} ("Active Cell:Active Cell"), "Row"=w901, "Column"=1) -> (w896:T4)
          n349 = property class="Tbl (strict)"(reference=w900, "Active Cell"=w896) -> (reference out=w899:refnum<vi>)  [unwired: 1 in, 1 out]
          n350 = Select(t=u32 65280 ("Active Cell:Cell Background Color"), s=w892, f=u32 16711680 ("Active Cell:Cell Background Color")) -> (s? t:f=w898:u32)
          n351 = property class="Tbl (strict)"(reference=w899, "Cell BG Color"=w898) -> ()  [unwired: 1 in, 2 out]
          n352 = Number To Fractional String(number=w906, precision (6)=i16 3) -> (F-format string=w897:string)  [unwired: 2 out]
        }
        n353 = property class="Tbl (strict)"(reference=w881) -> (reference out=w883:refnum<vi>, "Value"=w882:string[][])  [unwired: 1 in, 1 out]
        n354 = Replace Array Subset(array=w882, new element=w886, index (col)=1 ("disabled index (col)")) -> (w885:string[][])  [unwired: 1 in]
        n355 = property class="Tbl (strict)"(reference=w883, "Value"=w885) -> ()  [unwired: 1 in, 2 out]
      }
      frame #15 {
        w922 = u8[] [25, 26]  # ADC Ch#
        n356 = for {
          tunnel: w922 -> [w940] mode=indexing
          tunnel: w921 -> [w941]
          tunnel: w920 -> [w939]
          tunnel: w913 -> [w931]
          tunnel: [w928] -> w918 mode=indexing
          tunnel: w916 -> [w926]
          shift-right: [w924] -> w911
          shift-left: TRUE -> [w925]
          i -> [w932]
          n357 = call "_Remote Calculate ADC.vi"("ADC Table"=w939, "Unit"=w926, "ADC Channel (64)"=w940, "ADC Values"=w941) -> ("In Range?"=w923:bool, "User Value"=w937:dbl)  [unwired: 2 out]
          n358 = And(x=w923, y=w925) -> (x .and. y?=w924:bool)
          n359 = Bundle By Name(cluster=T4 {"Row"=0, "Column"=0} ("Active Cell:Active Cell"), "Row"=w932, "Column"=1) -> (w927:T4)
          n360 = property class="Tbl (strict)"(reference=w931, "Active Cell"=w927) -> (reference out=w930:refnum<vi>)  [unwired: 1 in, 1 out]
          n361 = Select(t=u32 65280 ("Active Cell:Cell Background Color"), s=w923, f=u32 16711680 ("Active Cell:Cell Background Color")) -> (s? t:f=w929:u32)
          n362 = property class="Tbl (strict)"(reference=w930, "Cell BG Color"=w929) -> ()  [unwired: 1 in, 2 out]
          n363 = Number To Fractional String(number=w937, precision (6)=i16 3) -> (F-format string=w928:string)  [unwired: 2 out]
        }
        n364 = property class="Tbl (strict)"(reference=w913) -> (reference out=w915:refnum<vi>, "Value"=w914:string[][])  [unwired: 1 in, 1 out]
        n365 = Replace Array Subset(array=w914, new element=w918, index (col)=1 ("disabled index (col)")) -> (w917:string[][])  [unwired: 1 in]
        n366 = property class="Tbl (strict)"(reference=w915, "Value"=w917) -> ()  [unwired: 1 in, 2 out]
      }
      frame #16 {
        # "Heater"
        # "Gas Flow"
        n367 = property class="Clust (strict)"(reference=w958) -> ("Controls[]"=w959:refnum<vi>[])  [unwired: 1 in, 2 out]
        n368 = Boolean To (0,1)(Boolean=w952) -> (0, 1=w951:i16[])
        n369 = Boolean To (0,1)(Boolean=w955) -> (0, 1=w950:i16[])
        n370 = Index Array(array=w950) -> (element #2=w949:i16, element #3=w945:i16)  [unwired: 3 in, 1 out]
        n371 = Index Array(array=w951, index #1=2 ("index"), index #2=4 ("index")) -> (element #1=w948:i16, element #2=w944:i16)
        n372 = Add(x=w948, y=w949) -> (x+y=w947:i16)
        n373 = Add(x=w944, y=w945) -> (x+y=w943:i16)
        n374 = Index Array(array=w959) -> (element #1=w954:refnum<vi>, element #2=w953:refnum<vi>)  [unwired: 2 in]
        n375 = To Variant(anything=w947) -> (Variant=w946:variant)
        n376 = To Variant(anything=w943) -> (Variant=w942:variant)
        n377 = property class="Ctl"(reference=w954, "Value"=w946) -> ()  [unwired: 1 in, 2 out]
        n378 = property class="Ctl"(reference=w953, "Value"=w942) -> ()  [unwired: 1 in, 2 out]
      }
    }
    n379 = Compound Arithmetic op=AND(w8, w6, w5, w4) -> (→"DC OK":bool)
    n380 = Compound Arithmetic op=AND(w55, w54, w53, w52, w51) -> (→"SVG OK":bool)
    n381 = Compound Arithmetic op=AND(w24, w17, w65, w64, w63, w62, w12) -> (→"Voltage OK":bool)
  }
